vi "Read 1D U32.vi"(7 "count (-1: rest)":i64=-1 format="%d elements", 8 "error in (no error)":errorcluster, 9 "offset (0)":u64 format="%d bytes", 10 "buffer in":u32[](array[numeric]), 11 "Pointer in":refnum<class "Pointer.lvclass">) -> (0 "error out":errorcluster, 1 "offset out":u64 format="%d bytes", 2 "buffer out":u32[](array[numeric]), 3 "Pointer out":refnum<class "Pointer.lvclass">)   [LabVIEW 2020, in "Memory Manager.lvlib" / "Pointer.lvclass"]
doc: "Reads <b>count</b> elements from the address specified by <b>pointer + offset</b> into the provided <b>buffer</b>."
uses:
  Pointer.lvclass
  Read (No Check) 1D U32.vi
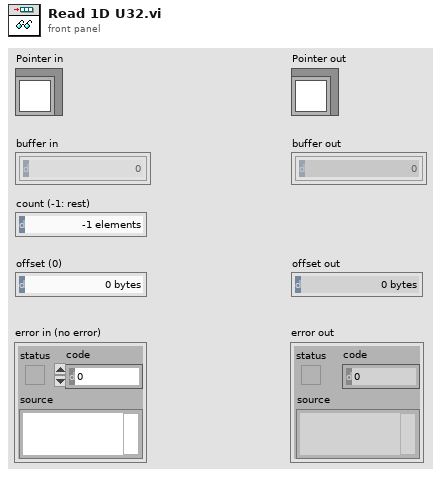
[diagram p1: front panel]
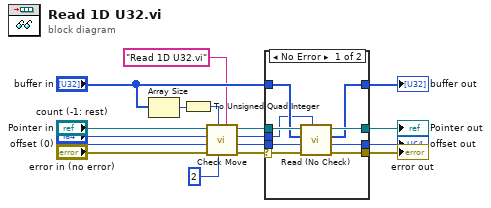
[diagram p0: block diagram]
diagram:
  n1 = Array Size(array="buffer in") -> (size(s)=w13:i32)
  n2 = To Unsigned Quad Integer(1:w13) -> (0:w7:u64)
  n3 = call "Check Move.vi"("source vi name"="Read 1D U32.vi", "count power of 2"=i16 2, "buffer count"=w7, "error in (no error)"="error in (no error)", "offset (0)"="offset (0)", "move count (-1: rest)"="count (-1: rest)", "Pointer in"="Pointer in") -> ("error out"=w10:errorcluster, "offset"=w9:u64, "count"=w8:u64, "Pointer out"=w11:refnum<class "Pointer.lvclass">)  [unwired: 1 in]
  n4 = case shown="No Error" w10 {
    selector: w10 -> [w26 w29]
    tunnel: w11 -> [w24 w28]
    tunnel: w9 -> [w25 w30]
    tunnel: "buffer in" -> [w19 w27]
    tunnel: [w23 w29] -> w17
    tunnel: [w22 w28] -> w15
    tunnel: [w21 w30] -> w14
    tunnel: [w20 w27] -> w16
    tunnel: w8 -> [w18 _]
    frame No Error {
      n5 = call-poly "Read (No Check).vi"("count"=w18, "error in (no error)"=w26, "offset (0)"=w25, "buffer in"=w19, "Pointer in"=w24) -> ("error out"=w23:errorcluster, "offset out"=w21:u64, "buffer out"=w20:u32[], "Pointer out"=w22:refnum<class "Pointer.lvclass">)  [unwired: 3 in]
    }
    frame Error {
    }
  }
  "error out" <- w17
  "Pointer out" <- w15
  "buffer out" <- w16
  "offset out" <- w14
